vi "Parse Xml Node Recursively.vi"(6 "VI Data":T1[](array[typedef]), 8 "error in":errorcluster, 9 "Parents":string[](array[string]), 10 "XML File Path":path, 11 "Node in":refnum<k20>) -> (0 "error out":errorcluster, 2 "VI Data out":T1[](array[typedef]), 3 "Node out":refnum<k20>)   [LabVIEW 2020, in "VI Properties Editor.lvlib"]
uses:
  VI Properties Editor.lvlib
  CTLs/XPath Get Attribute.ctl
  <vilib>/picture/picture.llb/imagedata.ctl
  CTLs/VI Properties.ctl
  CTLs/Control Properties.ctl
  CTLs/VI Data.ctl
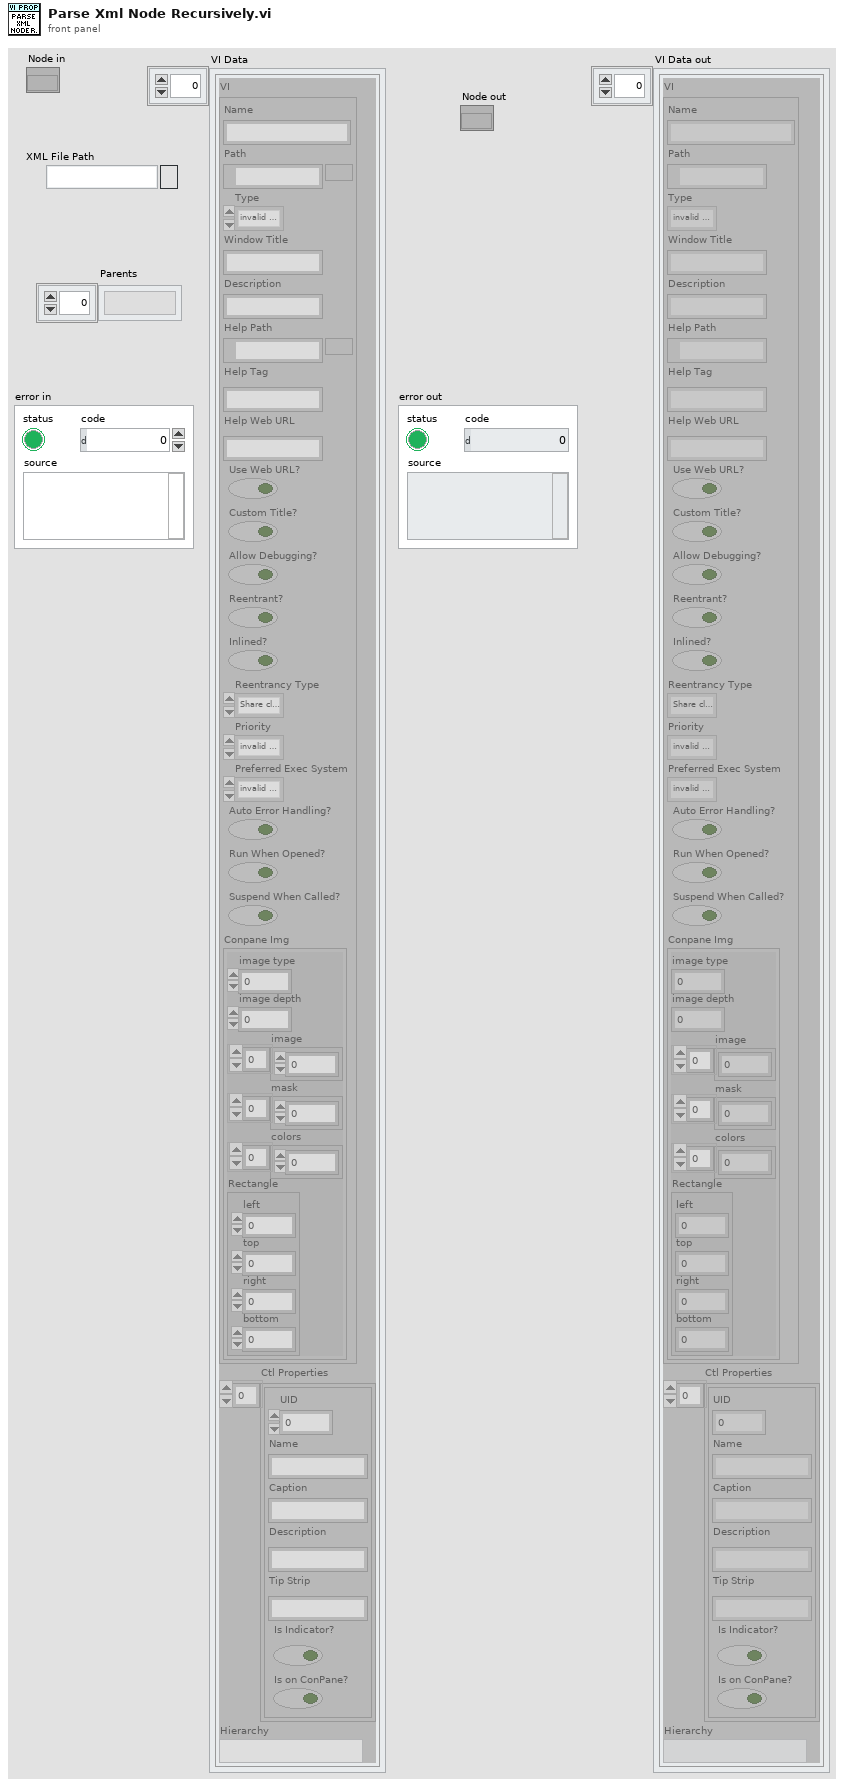
[diagram p1: front panel]
types:
  T1 = typedef "VI Properties Editor.lvlib/VI Data.ctl" = cluster{"VI":T2, "Ctl Properties":T4[], "Hierarchy":string}
  T2 = typedef "VI Properties Editor.lvlib/VI Properties.ctl" = cluster{"Name":string, "Path":path, "Type":enum32{"invalid VI type", "Standard VI", "Control VI", "Global VI", "Polymorphic VI", "Configuration VI", "SubSystem", "Facade VI", "Method VI", "Statechart Diagram VI"}, "Window Title":string, "Description":string, "Help Path":path, "Help Tag":string, "Help Web URL":string, "Use Web URL?":bool, "Custom Title?":bool, "Allow Debugging?":bool, "Reentrant?":bool, "Inlined?":bool, "Reentrancy Type":enum16{"Share clones between instances", "Preallocate clone for each instance"}, "Priority":enum32{"invalid priority", "background priority", "normal priority", "above normal priority", "high priority", "time critical priority", "subroutine"}, "Preferred Exec System":enum32{"invalid execution system", "user interface", "standard", "instrument i/o", "data acquisition", "other 1", "other 2", "same as caller"}, "Auto Error Handling?":bool, "Run When Opened?":bool, "Suspend When Called?":bool, "Conpane Img":T3}
  T3 = typedef "imagedata.ctl" = cluster{"image type":i32, "image depth":i32, "image":u8[], "mask":u8[], "colors":u32[], "Rectangle":cluster{"left":i16, "top":i16, "right":i16, "bottom":i16}}
  T4 = typedef "VI Properties Editor.lvlib/Control Properties.ctl" = cluster{"UID":i32, "Name":string, "Caption":string, "Description":string, "Tip Strip":string, "Is Indicator?":bool, "Is on ConPane?":bool}
  T5 = typedef "VI Properties Editor.lvlib/XPath Get Attribute.ctl" = enum16{"Item[@Type='VI']/@URL", "Item[@Type='LVClass']/@URL", "Item[@Type='Library']/@URL", "Item[@Type='Folder' and not (@URL)]/@Name", "@Name"}
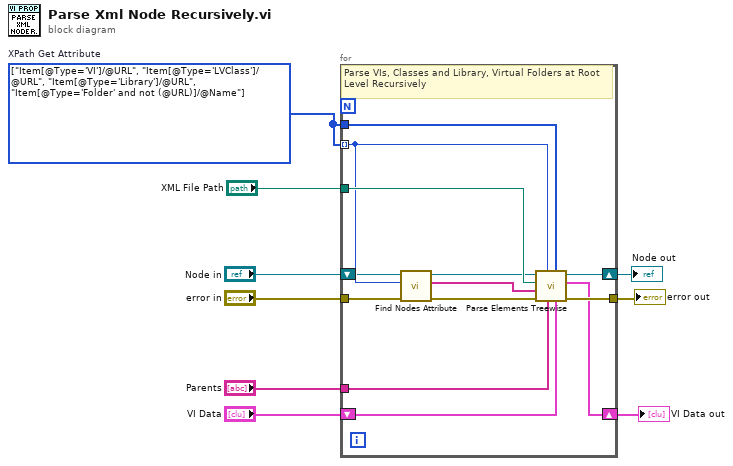
[diagram p0: block diagram]
diagram:
  w7 = T5[] [enum."Item[@Type='VI']/@URL", enum."Item[@Type='LVClass']/@URL", enum."Item[@Type='Library']/@URL", enum."Item[@Type='Folder' and not (@URL)]/@Name"] items=["Item[@Type='VI']/@URL", "Item[@Type='LVClass']/@URL", "Item[@Type='Library']/@URL", "Item[@Type='Folder' and not (@URL)]/@Name", "@Name"]  # XPath Get Attribute
  n1 = for {
    tunnel: "XML File Path" -> [w22]
    tunnel: [w21] -> w8
    tunnel: "error in" -> [w19]
    tunnel: "Parents" -> [w18]
    shift-right: [w10] -> w3
    shift-left: "VI Data" -> [w17]
    tunnel: w7 -> [w16] mode=indexing
    tunnel: w7 -> [w15]
    shift-right: [w11] -> w1
    shift-left: "Node in" -> [w14]
    # "Parse VIs, Classes and Library, Virtual Folders at Root Level Recursively"
    n2 = call "Find Nodes Attribute.vi"("error in"=w19, "XPath"=w16, "Node in"=w14) -> ("error out"=w20:errorcluster, "Attribute"=w13:string[], "Node out"=w12:refnum<k20>)  [unwired: 6 in]
    n3 = call "Parse Elements Treewise.vi"("VI Data in"=w17, "XPath Get Attribute"=w15, "Parents"=w18, "XPath Node Attribute"=w16, "error in"=w20, "Attribute"=w13, "XML File Path"=w22, "Node in"=w12) -> ("error out"=w21:errorcluster, "VI Data out"=w10:T1[], "Node out"=w11:refnum<k20>)  [unwired: 1 in]
  }
  "error out" <- w8
  "VI Data out" <- w3
  "Node out" <- w1
